vi "InjectChild.vi"(8 "error in (no error)":errorcluster, 10 "Child":refnum<class "Class.lvclass">, 11 "Class in":refnum<class "Class.lvclass">) -> (0 "error out":errorcluster, 3 "Class out":refnum<class "Class.lvclass">)   [LabVIEW 2020, in "Mermaid.lvlib" / "Class.lvclass"]
uses:
  Class.lvclass
  C:/Users/AdamMetcalf/Desktop/Mermaid/_iClass/iClass.lvclass
  Class.lvclass/Class.ctl
  C:/Users/AdamMetcalf/Desktop/Mermaid/_Class/Class.lvclass
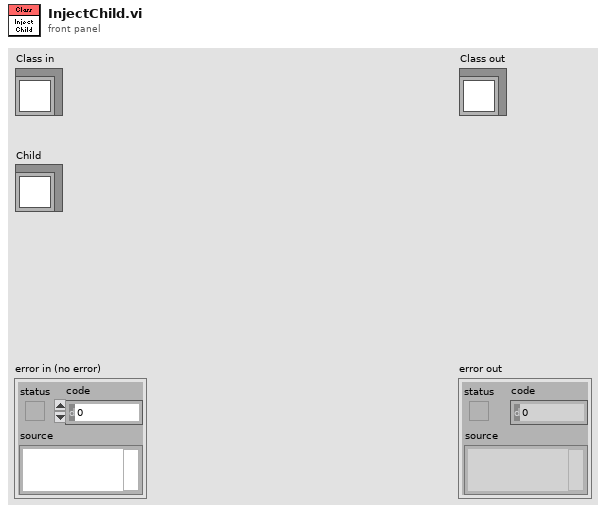
[diagram p1: front panel]
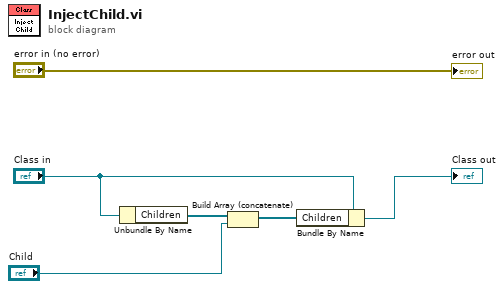
[diagram p0: block diagram]
diagram:
  n1 = Unbundle By Name("Class in") -> ("Children"=w5:refnum<class "iClass.lvclass">[])
  n2 = Build Array (concatenate)(w5, "Child") -> (w3:refnum<class "iClass.lvclass">[])
  n3 = Bundle By Name(cluster="Class in", "Children"=w3) -> (→"Class out":refnum<class "Class.lvclass">)
  "error out" <- "error in (no error)"
